vi "myRIOXC Pin Click.vi"(8 "error in":errorcluster, 9 "Pin Ref":refnum<vi>, 10 "Data In":bool[](array[boolean]), 11 "Connector Ref":refnum<vi>) -> (0 "error out":errorcluster, 1 "Value Change?":bool, 2 "Data Out":bool[](array[boolean]))   [LabVIEW 2021]
doc: "When user clicks a Pin, this VI decides whether the Pin value will be changed."
panel:
  # "When user clicks a Pin, this VI decides whether the Pin value will be changed."
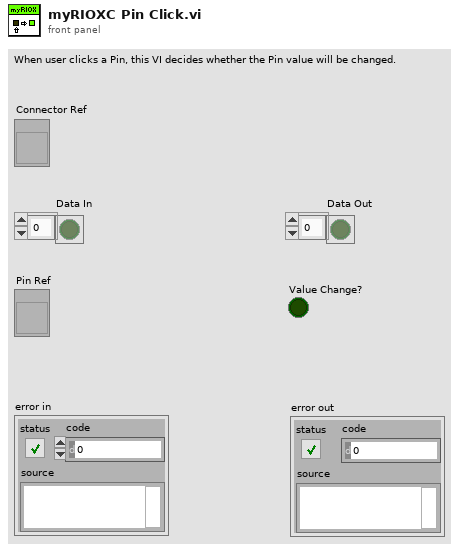
[diagram p1: front panel]
types:
  T1 = enum8{"Enabled", "Disabled", "Disabled and Grayed Out"}
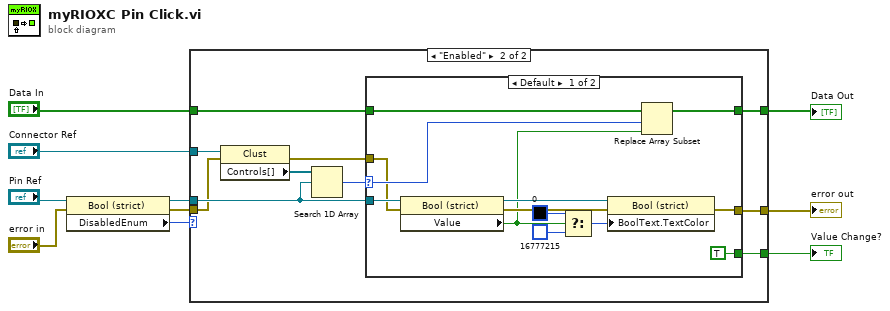
[diagram p0: block diagram]
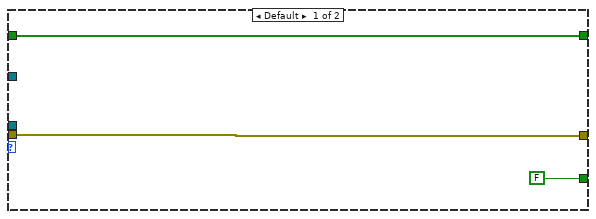
[diagram p2: hidden frame]
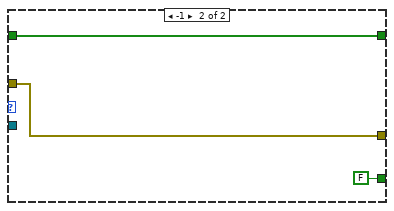
[diagram p3: hidden frame]
diagram:
  n1 = property class="Bool (strict)"(reference="Pin Ref", error in="error in") -> (reference out=w7:refnum<vi>, error out=w4:errorcluster, "DisabledEnum"=w1:T1)
  n2 = case shown="\"Enabled\"" w1 {
    tunnel: "Data In" -> [w13 w22]
    tunnel: w7 -> [_ w19]
    tunnel: [w13 w21] -> w5
    tunnel: [FALSE w14] -> w10
    tunnel: [w11 w20] -> w8
    tunnel: w4 -> [w11 w16]
    tunnel: "Connector Ref" -> [_ w18]
    frame Default {
    }
    frame "Enabled" {
      n3 = property class="Clust"(reference=w18, error in=w16) -> (error out=w15:errorcluster, "Controls[]"=w17:refnum<vi>[])  [unwired: 1 out]
      n4 = Search 1D Array(1D array=w17, element=w19) -> (index of element=w23:i32)  [unwired: 1 in]
      n5 = case shown="Default" w23 {
        selector: w23 -> [w34 _]
        tunnel: w22 -> [w36 w39]
        tunnel: [w35 w39] -> w21
        tunnel: [w29 w38] -> w20
        tunnel: w19 -> [w33 _]
        tunnel: w15 -> [w32 w38]
        tunnel: [TRUE FALSE] -> w14
        frame Default {
          n6 = property class="Bool (strict)"(reference=w33, error in=w32) -> (reference out=w31:refnum<vi>, error out=w30:errorcluster, "Value"=w28:bool)
          n7 = Select(t=u32 0, s=w28, f=u32 16777215) -> (s? t:f=w25:u32)
          n8 = property class="Bool (strict)"(reference=w31, error in=w30, "BoolText.TextColor"=w25) -> (error out=w29:errorcluster)  [unwired: 1 out]
          n9 = Replace Array Subset(array=w36, new element=w28, index=w34) -> (w35:bool[])
        }
        frame -1 {
        }
      }
    }
  }
  "Value Change?" <- w10
  "error out" <- w8
  "Data Out" <- w5
